vi "Dummy_Device.vi"(7 "Device-specific in":variant, 8 "error in (no error)":errorcluster, 10 "Position in":dbl[](array[numeric]), 11 "Operation":T2(ring)) -> (0 "error out":errorcluster, 1 "Device properties":cluster{"Axes":string[], "Tolerance":dbl[][]}, 2 "Position out":dbl[](array[numeric]), 3 "Status":T1, 5 "Device-specific out":variant)   [LabVIEW 2018]
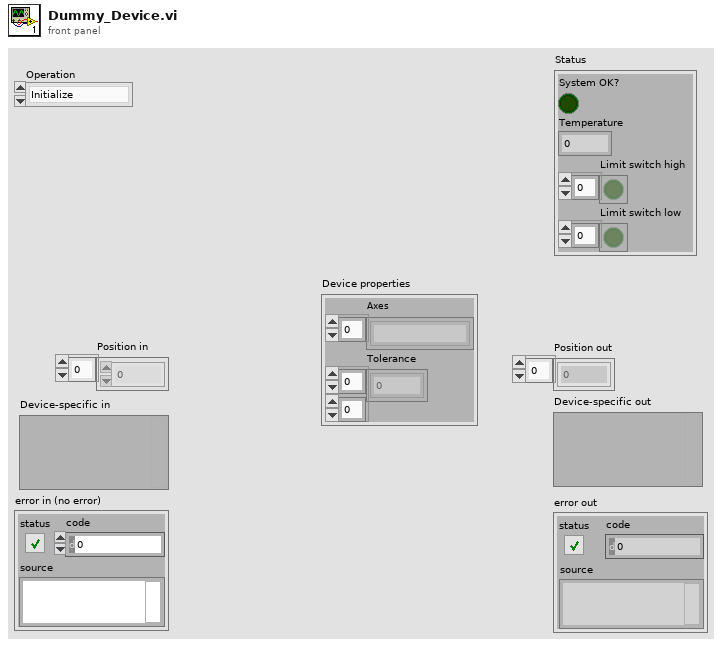
[diagram p1: front panel]
types:
  T1 = cluster{"System OK?":bool, "Temperature":dbl, "Limit switch high":bool[], "Limit switch low":bool[]}
  T2 = enum16{"Initialize", "Shut down", "Set position", "Get position", "Get status", "Other settings"}
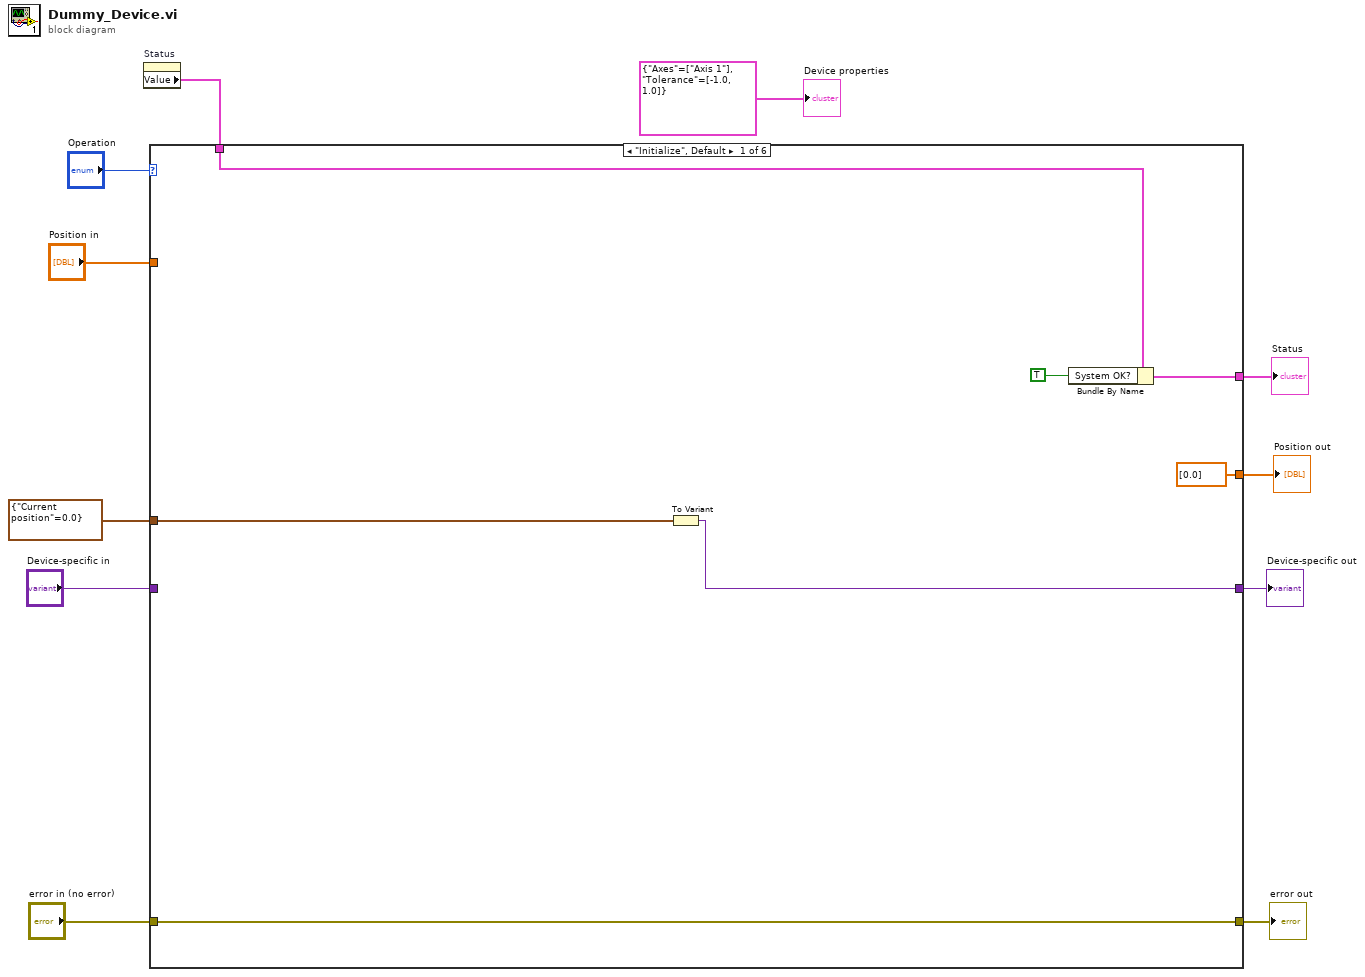
[diagram p0: block diagram]
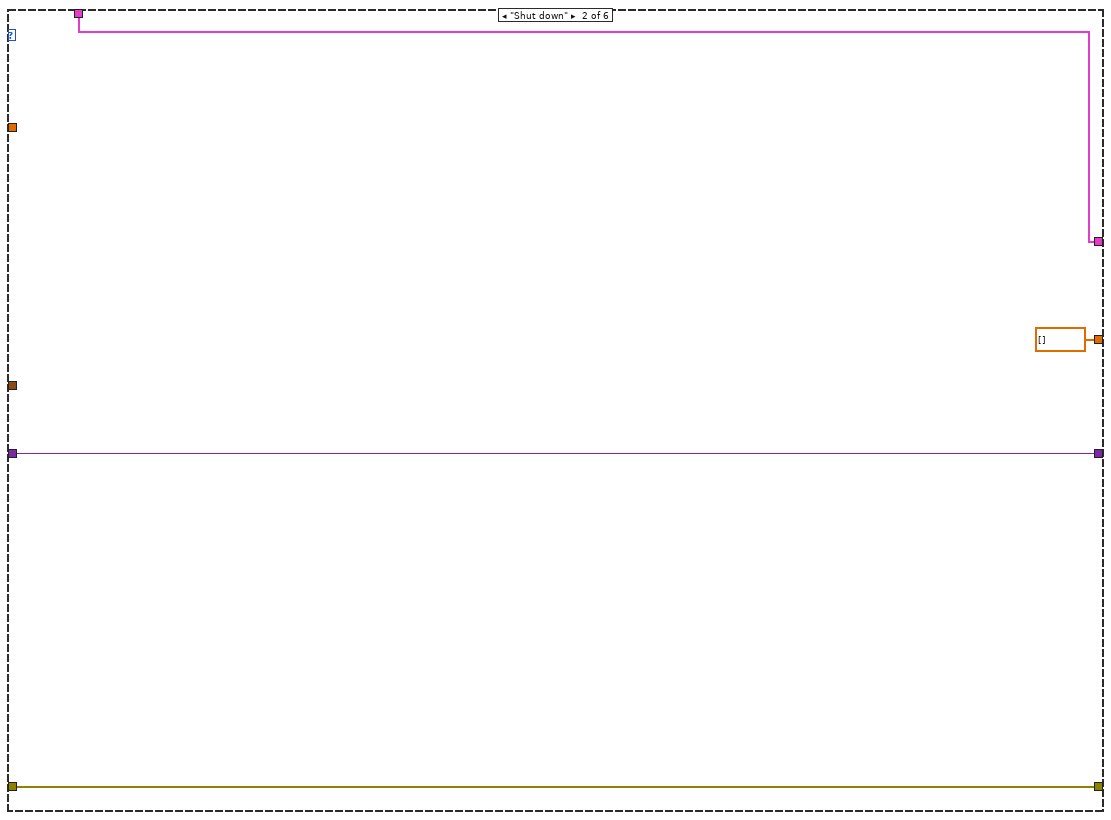
[diagram p2: hidden frame]
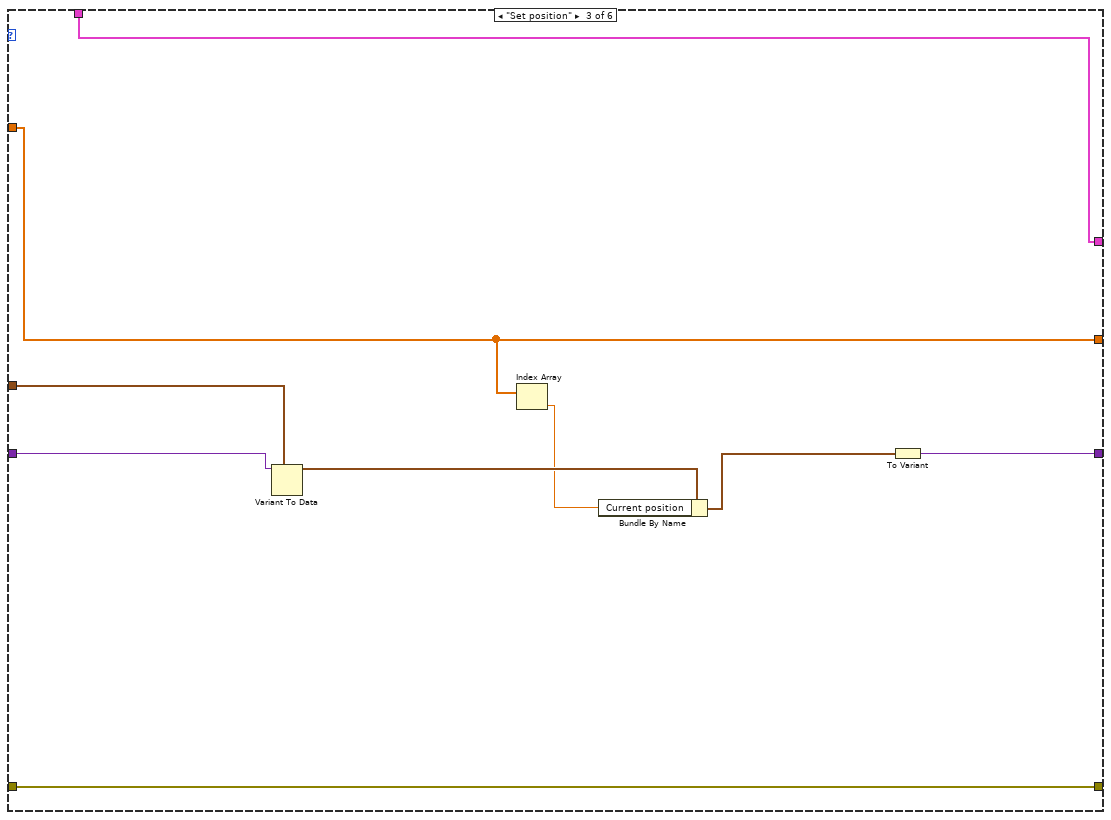
[diagram p3: hidden frame]
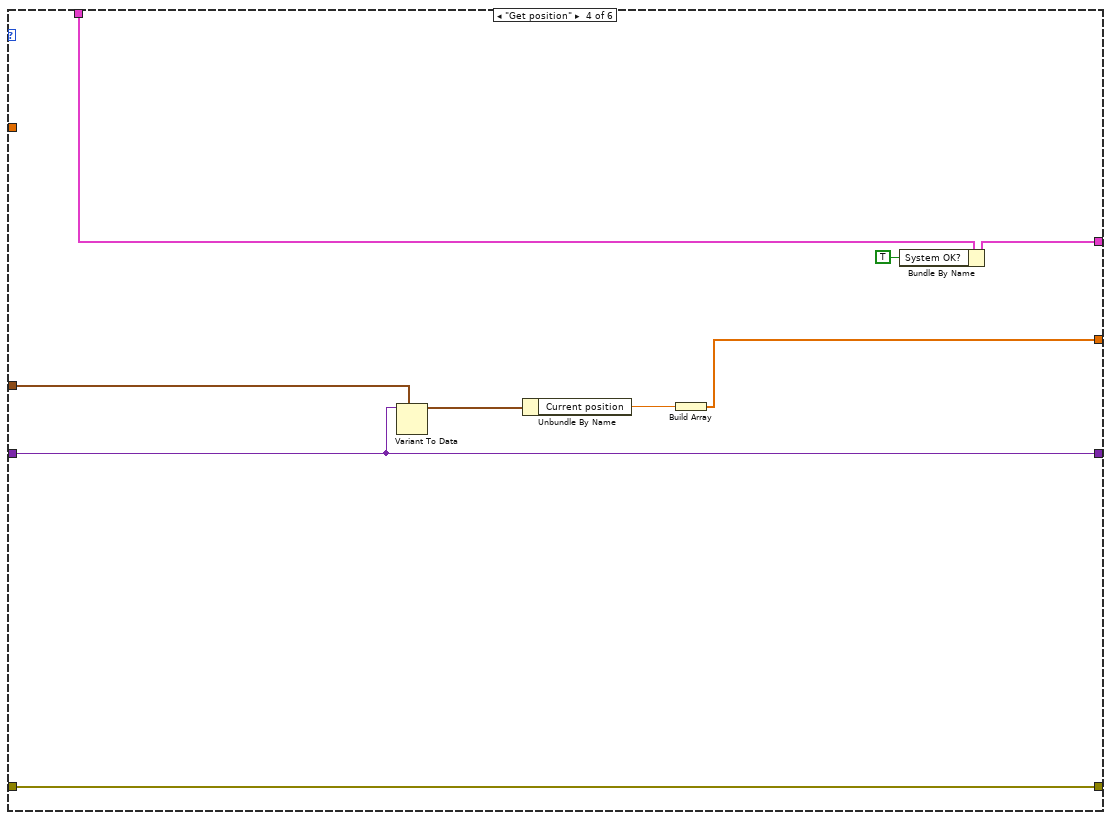
[diagram p4: hidden frame]
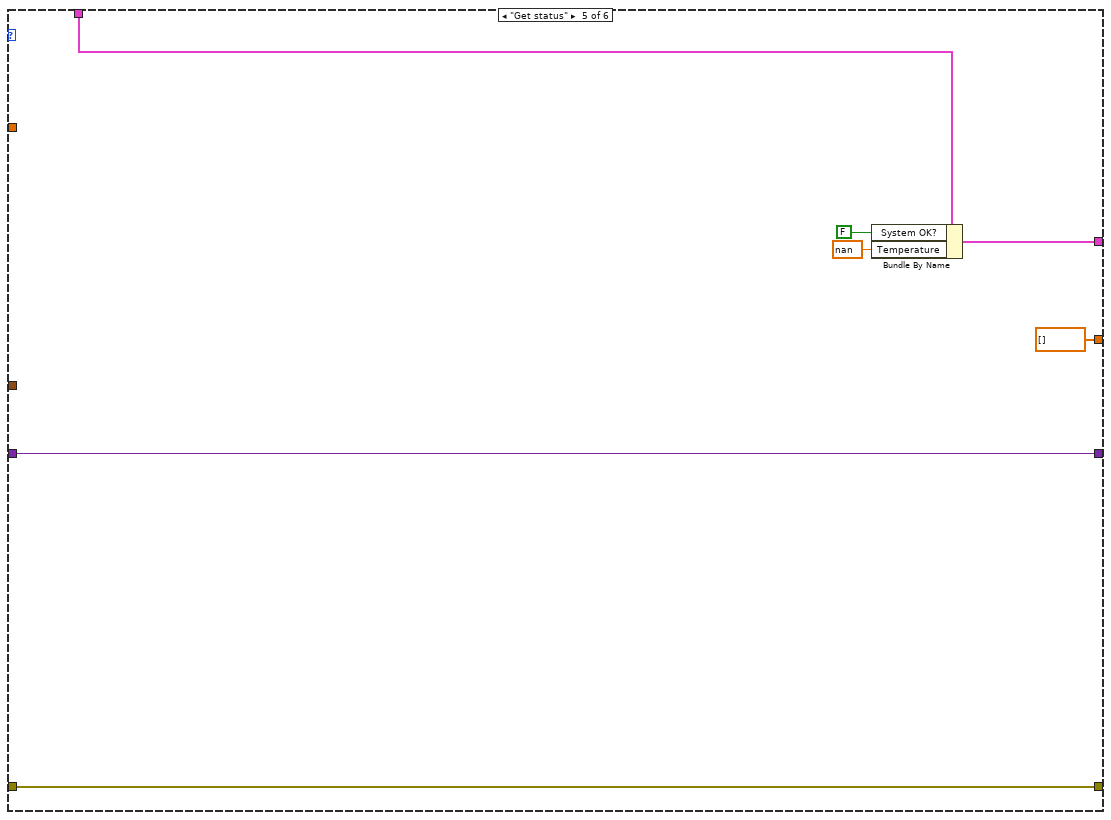
[diagram p5: hidden frame]
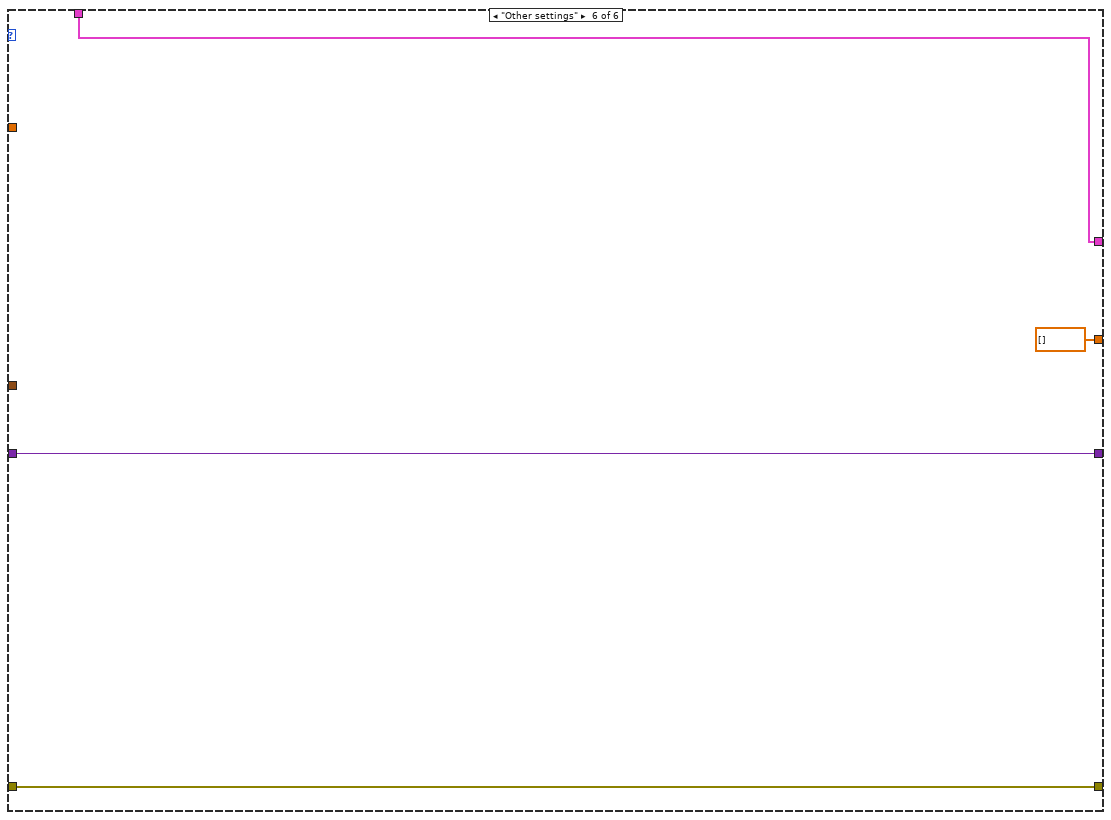
[diagram p6: hidden frame]
diagram:
  n1 = property on="Status" class="Clust (strict)"() -> ("Value"=w10:T1)  [unwired: 2 in, 2 out]
  n2 = case shown="\"Initialize\", Default" "Operation" {
    tunnel: "Position in" -> [_ _ w26 _ _ _]
    tunnel: w10 -> [w18 w22 w31 w40 w47 w51]
    tunnel: [w17 w22 w31 w38 w46 w51] -> w9
    tunnel: "Device-specific in" -> [_ w21 w29 w36 w43 w50]
    tunnel: [dbl[] [0.0] ("Position in") dbl[] [] ("Position in") w26 w32 dbl[] [] ("Position in") dbl[] [] ("Position in")] -> w6
    tunnel: [w12 w21 w23 w36 w43 w50] -> w5
    tunnel: [w15 w20 w30 w39 w42 w49] -> w4
    tunnel: "error in (no error)" -> [w15 w20 w30 w39 w42 w49]
    tunnel: cluster{"Current position":dbl} {"Current position"=0.0} -> [w13 _ w28 w35 _ _]
    frame "Initialize", Default {
      n3 = To Variant(anything=w13) -> (Variant=w12:variant)
      n4 = Bundle By Name(cluster=w18, "System OK?"=TRUE) -> (w17:T1)
    }
    frame "Shut down" {
    }
    frame "Set position" {
      n5 = Variant To Data(type=w28, Variant=w29) -> (data=w27:cluster{"Current position":dbl})  [unwired: 1 in, 1 out]
      n6 = Index Array(array=w26) -> (element=w25:dbl)  [unwired: 1 in]
      n7 = Bundle By Name(cluster=w27, "Current position"=w25) -> (w24:cluster{"Current position":dbl})
      n8 = To Variant(anything=w24) -> (Variant=w23:variant)
    }
    frame "Get position" {
      n9 = Variant To Data(type=w35, Variant=w36) -> (data=w34:cluster{"Current position":dbl})  [unwired: 1 in, 1 out]
      n10 = Unbundle By Name(w34) -> ("Current position"=w33:dbl)
      n11 = Build Array(w33) -> (w32:dbl[])
      n12 = Bundle By Name(cluster=w40, "System OK?"=TRUE) -> (w38:T1)
    }
    frame "Get status" {
      n13 = Bundle By Name(cluster=w47, "System OK?"=FALSE, "Temperature"=nan) -> (w46:T1)
    }
    frame "Other settings" {
    }
  }
  "Status" <- w9
  "Device-specific out" <- w5
  "error out" <- w4
  "Position out" <- w6
  "Device properties" <- cluster{"Axes":string[], "Tolerance":dbl[][]} {"Axes"=["Axis 1"], "Tolerance"=[[-1.0, 1.0]]} ("Device properties")
